vi "Temperatura.vi"(1 "Aviso temperatura":string) -> (0 "String":string)   [LabVIEW 2015]
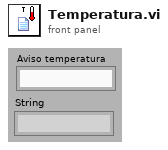
[diagram p1: front panel]
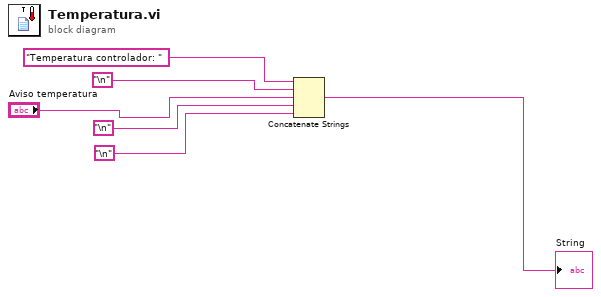
[diagram p0: block diagram]
diagram:
  n1 = Concatenate Strings("Temperatura controlador: ", "\n", "Aviso temperatura", "\n", "\n") -> (→"String":string)
